vi "Configure Histogram.vi"(0 "VISA resource name":refnum<visa-resource-name>, 1 "Histogram Orientation (0: Horizontal)":i32(ring) items=["Horizontal", "Vertical"], 2 "Histogram Top (5)":dbl, 3 "Histogram Left (100E-9)":dbl, 5 "Histogram Source (1: Channel 1)":i32(ring) items=["Channel 1", "Channel 2", "Channel 3", "Channel 4", "Function 1", "Function 2", "Function 3", "Function 4", "Memory 1", "Memory 2", "Memory 3", "Memory 4"], 7 "Histogram Mode (0: Off)":i32(ring) items=["Off", "Waveforms", "Measurement"], 9 "Histogram Size (4.0)":dbl, 11 "error in (no error)":errorcluster, 12 "Histogram Right (900E-9)":dbl, 13 "Histogram Bottom (-1)":dbl) -> (4 "VISA resource name out":refnum<visa-resource-name>, 15 "error out":errorcluster)   [LabVIEW 2009, in "Agilent 8000 Series.lvlib"]
doc: "Configures the Histogram properties of an oscilloscope. You can configure the Histogram Type, Histogram Size and so on."
uses:
  Agilent 8000 Series.lvlib
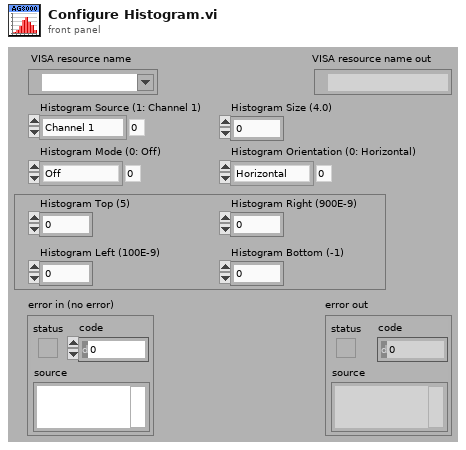
[diagram p1: front panel]
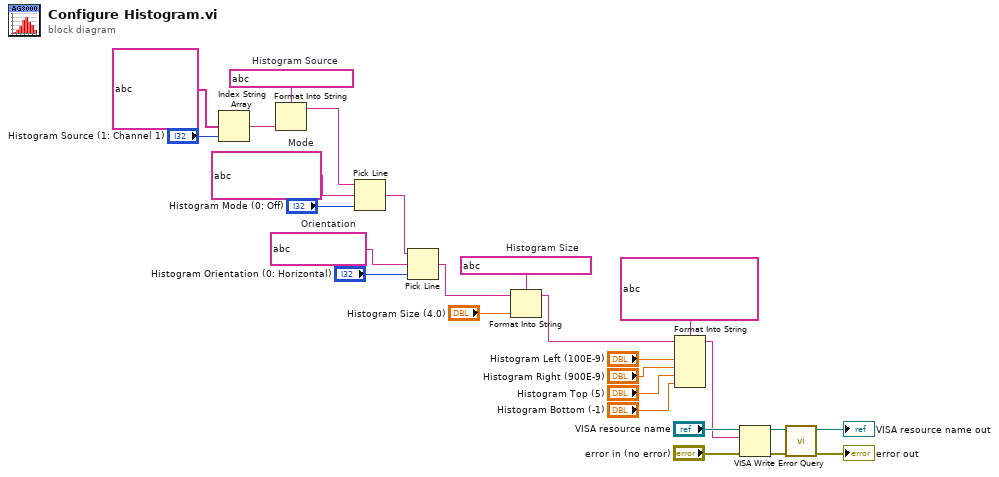
[diagram p0: block diagram]
diagram:
  w11 = string ?  # Histogram Size
  w13 = string ?  # Orientation
  w16 = string ?  # Mode
  w18 = string ?  # Histogram Source
  n1 = Index String Array(1:"Histogram Source (1: Channel 1)", 2:string[] ?) -> (0:w19:string)  [unwired: 1 in]
  n2 = Format Into String(format string=w18, w19) -> (resulting string=w15:string)  [unwired: 2 in, 1 out]
  n3 = Pick Line(string ("")=w15, multi-line string=w16, line index="Histogram Mode (0: Off)") -> (output string=w12:string)
  n4 = Pick Line(string ("")=w12, multi-line string=w13, line index="Histogram Orientation (0: Horizontal)") -> (output string=w9:string)
  n5 = Format Into String(format string=w11, initial string=w9, "Histogram Size (4.0)") -> (resulting string=w6:string)  [unwired: 1 in, 1 out]
  n6 = Format Into String(format string=string ?, initial string=w6, "Histogram Left (100E-9)", "Histogram Right (900E-9)", "Histogram Top (5)", "Histogram Bottom (-1)") -> (resulting string=w2:string)  [unwired: 1 in, 1 out]
  n7 = VISA Write(VISA resource name="VISA resource name", write buffer=w2, error in (no error)="error in (no error)") -> (VISA resource name out=w22:refnum<visa-resource-name>, error out=w21:errorcluster)  [unwired: 1 out]
  n8 = call "Error Query.vi"("error in (no error)"=w21, "VISA resource name"=w22) -> ("error out"=→"error out":errorcluster, "VISA resource name out"=→"VISA resource name out":refnum<visa-resource-name>)  [unwired: 6 in, 2 out]
